vi "Wait on Notification.vi"(8 "error in (no error)":errorcluster, 9 "timeout in ms (-1)":i32=-1, 11 "NotifierMessenger in":refnum<class "NotifierMessenger.lvclass">) -> (0 "error out":errorcluster, 1 "timed out?":bool, 2 "Message":refnum<class "MSG.lvclass">, 3 "NotifierMessenger out":refnum<class "NotifierMessenger.lvclass">)   [LabVIEW 2011, in "Messenging.lvlib" / "NotifierMessenger.lvclass"]
uses:
  NotifierMessenger.lvclass
  TextVarientMessage/MSG.lvclass
  NotifierMessenger.lvclass/NotifierMessenger.ctl
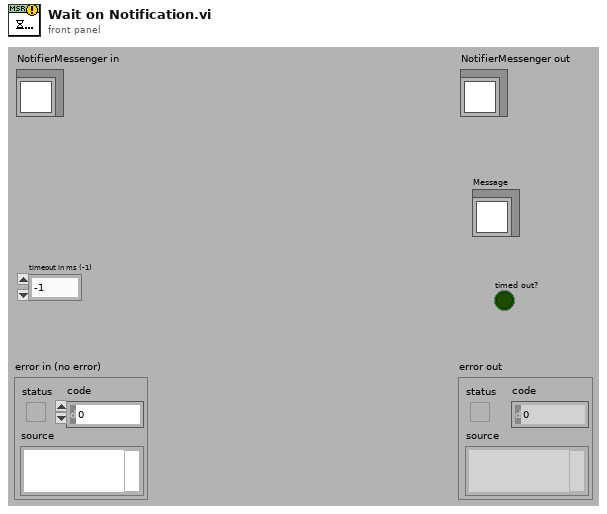
[diagram p1: front panel]
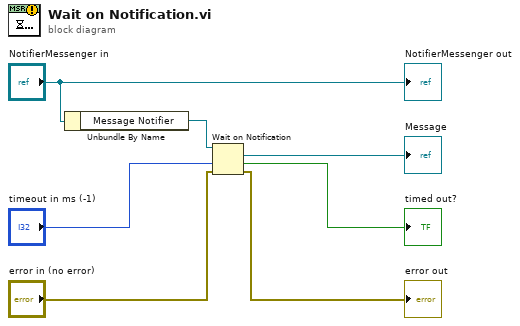
[diagram p0: block diagram]
diagram:
  n1 = Unbundle By Name("NotifierMessenger in") -> ("Message Notifier"=w6:refnum<notifier>)
  n2 = Wait on Notification(notifier=w6, timeout in ms (-1)="timeout in ms (-1)", error in (no error)="error in (no error)") -> (notification=→"Message":refnum<class "MSG.lvclass">, timed out?=→"timed out?":bool, error out=→"error out":errorcluster)  [unwired: 2 out]
  "NotifierMessenger out" <- "NotifierMessenger in"
